vi "qp_take AS step.vi"(8 "P(k)":dbl[](array[numeric]), 9 "X(k)":dbl[](array[numeric]), 10 "b not working set":dbl[](array[numeric]), 11 "A not working set":T1) -> (1 "X(k+1)":dbl[](array[numeric]), 2 "blocking index":i32, 3 "stepsize":dbl)   [LabVIEW 2017, in "NI_Gmath.lvlib"]
uses:
  <vilib>/gmath/NI_Gmath.lvlib
  <vilib>/Analysis/Matrix/Datatypes/RealMatrix.ctl
  <vilib>/Analysis/baseanly.llb/A x Vector.vi
  <vilib>/Analysis/NI_AALBase.lvlib
  <vilib>/Analysis/Matrix/NI_Matrix.lvlib
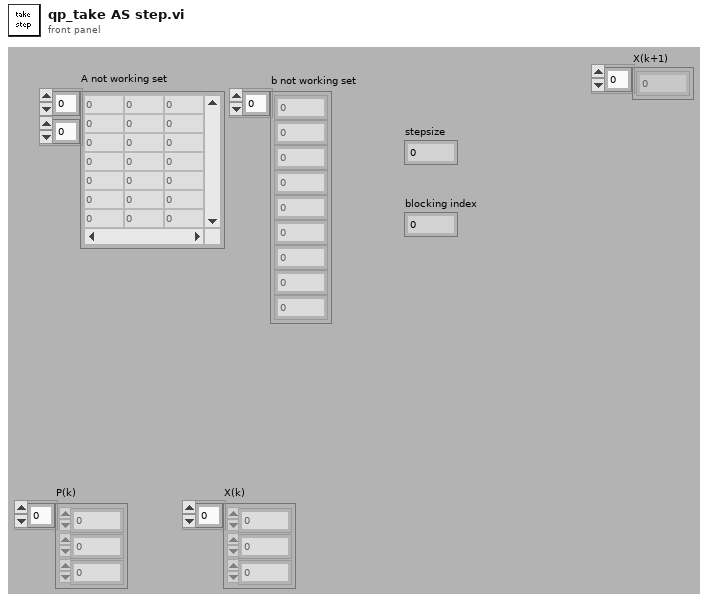
[diagram p1: front panel]
types:
  T1 = typedef "NI_Matrix.lvlib/RealMatrix.ctl" = dbl[][]
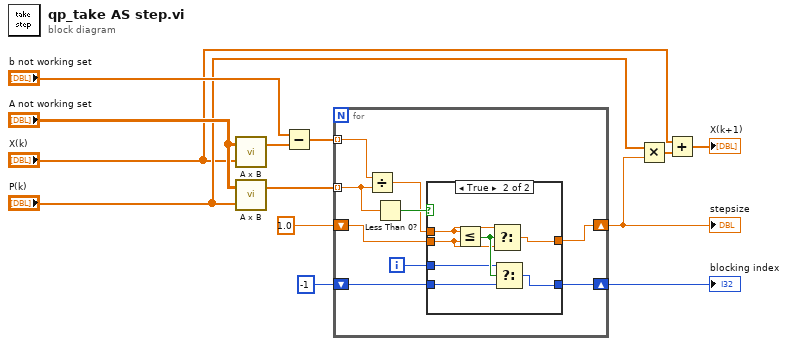
[diagram p0: block diagram]
diagram:
  n1 = call-poly <vilib>:"A x B.vi"("Vector"="X(k)", "A"="A not working set") -> ("A x Vector"=w11:dbl[])  [unwired: 1 out]
  n2 = call-poly <vilib>:"A x B.vi"("Vector"="P(k)", "A"="A not working set") -> ("A x Vector"=w6:dbl[])  [unwired: 1 out]
  n3 = Subtract(x="b not working set", y=w11) -> (x-y=w10:dbl[])
  n4 = for {
    tunnel: w10 -> [w15] mode=indexing
    tunnel: w6 -> [w18] mode=indexing
    shift-right: [w20] -> w5
    shift-left: 1.0 -> [w21]
    shift-right: [w14] -> w7
    shift-left: -1 -> [w16]
    i -> [w17]
    n5 = Divide(x=w15, y=w18) -> (x/y=w19:dbl)
    n6 = Less Than 0?(x=w18) -> (x < 0?=w22:bool)
    n7 = case shown="True" w22 {
      tunnel: w16 -> [w24 w25]
      tunnel: [w24 w28] -> w14
      tunnel: w21 -> [w23 w30]
      tunnel: [w23 w27] -> w20
      tunnel: w19 -> [_ w29]
      tunnel: w17 -> [_ w26]
      frame False {
      }
      frame True {
        n8 = Less Or Equal?(x=w29, y=w30) -> (x <= y?=w31:bool)
        n9 = Select(t=w29, s=w31, f=w30) -> (s? t:f=w27:dbl)
        n10 = Select(t=w26, s=w31, f=w25) -> (s? t:f=w28:i32)
      }
    }
  }
  "stepsize" <- w5
  "blocking index" <- w7
  n11 = Multiply(x="P(k)", y=w5) -> (x*y=w3:dbl[])
  n12 = Add(x="X(k)", y=w3) -> (x+y=→"X(k+1)":dbl[])
